vi "Test P Class.vi"() -> ()   [LabVIEW 2014, in "Alicat.lvlib"]
uses:
  Alicat.lvlib
  AlicatCommBank.lvclass
  Alicat.lvclass
  Controls/Gas.ctl
  Controls/CtlSetup.ctl
  Data/P/AlicatPData.lvclass
  P/P.lvclass
  Data/MC/AlicatMCData.lvclass
panel:
  out "SystemData 2":T1
  out "SystemData":T1
  out "DataOut":cluster{"P":dbl, "dP":dbl, "Q":dbl}
  in  "Boolean":bool
  out "error out":errorcluster
  in  "error in":errorcluster
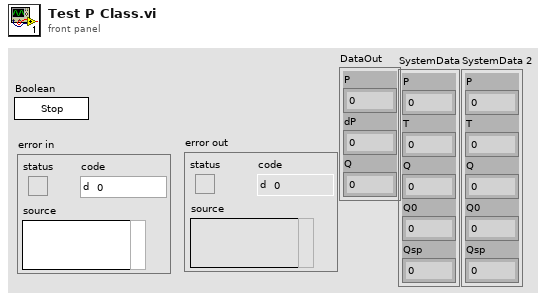
[diagram p1: front panel]
types:
  T1 = cluster{"P":sgl, "T":sgl, "Q":sgl, "Q0":sgl, "Qsp":sgl}
  T2 = typedef "Alicat.lvlib/Alicat.lvclass/CtlSetup.ctl" = cluster{"Name":string, "Address":string, "fullScale":dbl, "Gas":T3}
  T3 = typedef "Alicat.lvlib/Alicat.lvclass/Gas.ctl" = enum16{"Air", "Ar", "CH4", "CO", "CO2", "C2H6", "H2", "He", "N2", "NO", "Ne", "O2", "C3H8", "n-C4H10", "C2H2", "C2H4", "i-C2H10", "Kr", "Xe"}
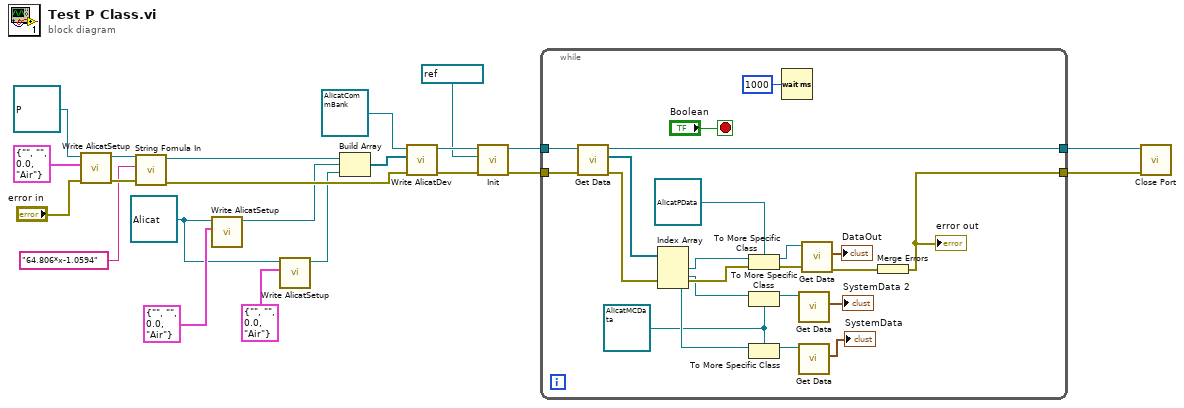
[diagram p0: block diagram]
diagram:
  w4 = refnum<class "Alicat.lvclass"> refnum ("Alicat")
  n1 = call "Write AlicatSetup.vi"("error in"="error in", "AlicatSetup"=T2 {"Name"="", "Address"="", "fullScale"=0.0, "Gas"=enum."Air"}, "Alicat in"=refnum<class "P.lvclass"> refnum ("Alicat_P in")) -> ("error out"=w11:errorcluster, "Alicat out"=w12:refnum<class "P.lvclass">)  [unwired: 7 in]
  n2 = call "String Fomula In.vi"("error in"=w11, "formula"="64.806*x-1.0594", "Alicat_P in"=w12) -> ("error out"=w9:errorcluster, "Alicat_P out"=w10:refnum<class "P.lvclass">)  [unwired: 7 in]
  n3 = call "Write AlicatSetup.vi"("AlicatSetup"=T2 {"Name"="", "Address"="", "fullScale"=0.0, "Gas"=enum."Air"}, "Alicat in"=w4) -> ("Alicat out"=w1:refnum<class "Alicat.lvclass">)  [unwired: 8 in, 1 out]
  n4 = call "Write AlicatSetup.vi"("AlicatSetup"=T2 {"Name"="", "Address"="", "fullScale"=0.0, "Gas"=enum."Air"}, "Alicat in"=w4) -> ("Alicat out"=w2:refnum<class "Alicat.lvclass">)  [unwired: 8 in, 1 out]
  n5 = Build Array(w10, w1, w2) -> (w21:refnum<class "Alicat.lvclass">[])
  n6 = call "Write AlicatDev.vi"("error in"=w9, "AlicatDev"=w21, "AlicatCommBank in"=refnum<class "AlicatCommBank.lvclass"> refnum ("AlicatCommBank.lvclass")) -> ("error out"=w18:errorcluster, "AlicatCommBank out"=w19:refnum<class "AlicatCommBank.lvclass">)  [unwired: 7 in]
  n7 = call-dynamic "Init.vi"("error in"=w18, "Port"=refnum<visa-resource-name> "COM7", "AlicatCommBank in"=w19) -> ("error out"=w6:errorcluster, "AlicatCommBank out"=w7:refnum<class "AlicatCommBank.lvclass">)  [unwired: 7 in]
  n8 = while {
    tunnel: w7 -> [w42]
    tunnel: w6 -> [w41]
    tunnel: [w37] -> w15
    tunnel: [w36] -> w14
    stop <- "Boolean" stop-if-true
    w27 = refnum<class "AlicatMCData.lvclass"> refnum ("AlicatMCData.lvclass")
    n9 = call-dynamic "Get Data.vi"("error in"=w41, "AlicatCommBank in"=w42) -> ("error out"=w40:errorcluster, "DataOut"=w32:refnum<class "Data.lvclass">[], "AlicatCommBank out"=w36:refnum<class "AlicatCommBank.lvclass">)  [unwired: 7 in]
    n10 = Index Array(array=w32) -> (element #1=w31:refnum<class "Data.lvclass">, element #2=w29:refnum<class "Data.lvclass">, element #3=w28:refnum<class "Data.lvclass">)  [unwired: 3 in]
    n11 = To More Specific Class(target class=refnum<class "AlicatPData.lvclass"> refnum ("AlicatMData in"), reference=w31, error in=w40) -> (specific class reference=w34:refnum<class "AlicatPData.lvclass">, error out=w33:errorcluster)
    n12 = To More Specific Class(target class=w27, reference=w29) -> (specific class reference=w26:refnum<class "AlicatMCData.lvclass">)  [unwired: 1 in, 1 out]
    n13 = To More Specific Class(target class=w27, reference=w28) -> (specific class reference=w25:refnum<class "AlicatMCData.lvclass">)  [unwired: 1 in, 1 out]
    n14 = Wait (ms)(milliseconds to wait=u32 1000) -> ()  [unwired: 1 out]
    n15 = call "Get Data.vi"("AlicatMData in"=w26) -> ("SystemData"=→"SystemData 2":T1)  [unwired: 8 in, 2 out]
    n16 = call "Get Data.vi"("AlicatMData in"=w25) -> ("SystemData"=→"SystemData":T1)  [unwired: 8 in, 2 out]
    n17 = call "Get Data.vi"("error in"=w33, "AlicatPData in"=w34) -> ("error out"=w38:errorcluster, "DataOut"=→"DataOut":cluster{"P":dbl, "dP":dbl, "Q":dbl})  [unwired: 7 in, 1 out]
    n18 = Merge Errors(w38) -> (w37:errorcluster)
    "error out" <- w37
  }
  n19 = call-dynamic "Close Port.vi"("error in (no error)"=w15, "Serial IO in"=w14) -> ()  [unwired: 8 in, 2 out]
